vi "FPGA_Main.vi"() -> ()   [LabVIEW 2020]
uses:
  <vilib>/Platform/TimedLoop/XDataNode/timing_clust.ctl
  <vilib>/Platform/TimedLoop/XDataNode/nitl_modes.ctl
  <vilib>/Platform/TimedLoop/XDataNode/wakeup.ctl
  <vilib>/rvi/Emulation/niFpgaSctlEmulationGetInTimedLoop.vi
  <vilib>/rvi/Emulation/niFpgaEmulationReportErrorSimple.vi
  <vilib>/rvi/Emulation/niFpgaGetClockAttributes.vi
  <vilib>/rvi/Emulation/niFpgaCriticalErrorInLSC.vi
  <vilib>/rvi/eio/common/nirviEmuTemplateMethod_errors.vi
  <vilib>/platform/TimedLoop/XDataNode/XDataNode.xnode
  <vilib>/eio/EIONode/EIONode.xnode
  <vilib>/Platform/TimedLoop/XDataNode/XDNodeRunTimeDep.lvlib
panel:
  in  "ch3_frequency":fxp<+,32,0>=2.4999957531690598e-05
  in  "ch2_frequency":fxp<+,32,0>=2.4999957531690598e-05
  in  "ch1_frequency":fxp<+,32,0>=2.4999957531690598e-05
  in  "ch3_duty":fxp<+,32,0>=0.5
  in  "ch2_duty":fxp<+,32,0>=0.5
  in  "ch1_duty":fxp<+,32,0>=0.5
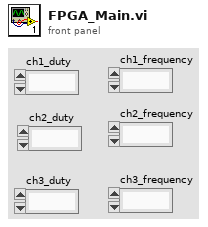
[diagram p1: front panel]
types:
  T1 = typedef "XDNodeRunTimeDep.lvlib/timing_clust.ctl" = cluster{"Expected End [f-1]":u64, "Actual End [f-1]":u64, "Finished Late? [f-1]":bool, "Expected End [i-1]":u64, "Actual End [i-1]":u64, "Finished Late? [i-1]":bool, "Expected Start [i]":u64, "Actual Start [i]":u64, "Expected Start [f]":u64, "Actual Start [f]":u64, "Source Name":string, "Structure Name":string, "Period":i64, "Deadline":i64, "Offset":i64, "Start":i64, "Priority":i32, "Timeout":i32, "Mode":T2, "Wakeup Reason":T3, "Error":errorcluster, "Source Type":string, "Secondary Source Type":string, "Global End Time":u64, "Global Start Time":u64, "Frame Duration":u64, "Iteration Duration":u64, "Assigned CPU":i32, "I/O Scan Engine Mode":u32}
  T2 = typedef "XDNodeRunTimeDep.lvlib/nitl_modes.ctl" = enum32{"No Change", "Process missed periods, maintain original phase", "Discard missed periods, maintain original phase", "Process missed periods, ignore original phase", "Discard missed periods, ignore original phase"}
  T3 = typedef "XDNodeRunTimeDep.lvlib/wakeup.ctl" = enum32{"Normal", "Aborted", "Asynchronous wakeup", "Timing source error", "Timed loop error", "Timeout"}
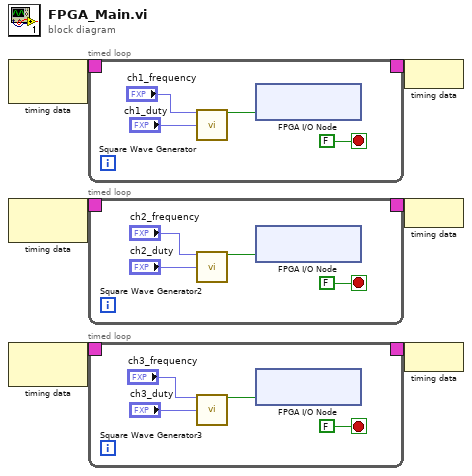
[diagram p0: block diagram]
diagram:
  n1 = node-c288() -> (w6:T1)  [unwired: 1 in]
  n2 = node-c288() -> (w4:T1)  [unwired: 1 in]
  n3 = node-c288() -> (w2:T1)  [unwired: 1 in]
  n4 = timed-loop {
    timing: w6 -> [_]
    timing-out: [_] -> w5
    stop <- FALSE stop-if-true
    n5 = call "Square Wave Generator"("frequency (periods/tick)"="ch1_frequency", "duty cycle (periods)"="ch1_duty") -> ("square wave out"=w8:bool)  [unwired: 13 in]
    n6 = xnode "FPGA I/O Node"("Mod1/DO0"=w8) -> ()  [unwired: 1 in, 1 out]
  }
  n7 = timed-loop {
    timing: w4 -> [_]
    timing-out: [_] -> w3
    stop <- FALSE stop-if-true
    n8 = call "Square Wave Generator2"("frequency (periods/tick)"="ch2_frequency", "duty cycle (periods)"="ch2_duty") -> ("square wave out"=w14:bool)  [unwired: 13 in]
    n9 = xnode "FPGA I/O Node"("Mod1/DO1"=w14) -> ()  [unwired: 1 in, 1 out]
  }
  n10 = timed-loop {
    timing: w2 -> [_]
    timing-out: [_] -> w1
    stop <- FALSE stop-if-true
    n11 = call "Square Wave Generator3"("frequency (periods/tick)"="ch3_frequency", "duty cycle (periods)"="ch3_duty") -> ("square wave out"=w20:bool)  [unwired: 13 in]
    n12 = xnode "FPGA I/O Node"("Mod1/DO2"=w20) -> ()  [unwired: 1 in, 1 out]
  }
  n13 = node-c288(w5) -> ()
  n14 = node-c288(w3) -> ()
  n15 = node-c288(w1) -> ()
